vi "Teleop Gears.vi"(11 "Joystick Data":T1) -> ()   [LabVIEW 2013]
uses:
  Joystick Data.ctl
  Gear state.ctl
  <vilib>/Rock Robotics/WPI/Solenoid/WPI_SolenoidValue.ctl
  <vilib>/Rock Robotics/WPI/Solenoid/WPI_SolenoidSetEnum.vi
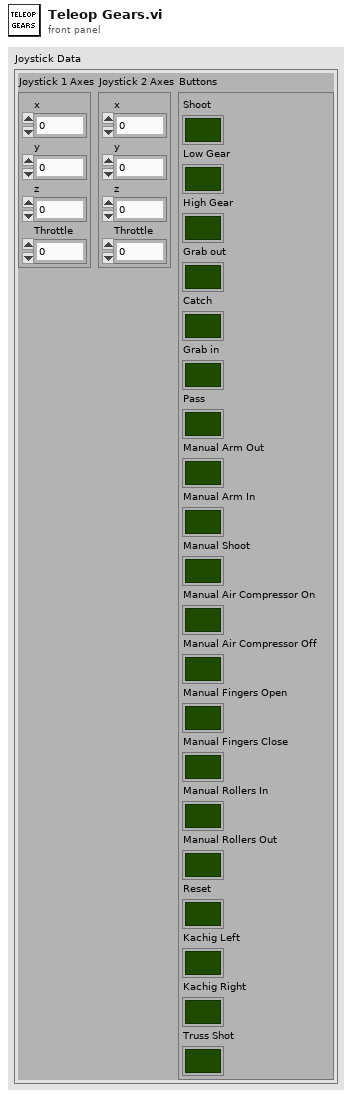
[diagram p1: front panel]
types:
  T1 = typedef "Joystick Data.ctl" = cluster{"Joystick 1 Axes":cluster{"x":dbl, "y":dbl, "z":dbl, "Throttle":dbl}, "Joystick 2 Axes":cluster{"x":dbl, "y":dbl, "z":dbl, "Throttle":dbl}, "Buttons":cluster{"Shoot":bool, "Low Gear":bool, "High Gear":bool, "Grab out":bool, "Catch":bool, "Grab in":bool, "Pass":bool, "Manual Arm Out":bool, "Manual Arm In":bool, "Manual Shoot":bool, "Manual Air Compressor On":bool, "Manual Air Compressor Off":bool, "Manual Fingers Open":bool, "Manual Fingers Close":bool, "Manual Rollers In":bool, "Manual Rollers Out":bool, "Reset":bool, "Kachig Left":bool, "Kachig Right":bool, "Truss Shot":bool}}
  T2 = typedef "Gear state.ctl" = enum16{"idle", "go to low gear", "go to high gear"}
  T3 = typedef "WPI_SolenoidDevRef.ctl" = cluster{"DevStatus":errorcluster, "Solenoid Module":T4, "Forward Solenoid Channel":T5, "Reverse Solenoid Channel":T5}
  T4 = typedef "FPGA_TypedefSolenoidModule.ctl" = enum16{"Solenoid Module 1", "Solenoid Module 2"}
  T5 = typedef "WPI_SolenoidChannel.ctl" = enum8{"Solenoid 1", "Solenoid 2", "Solenoid 3", "Solenoid 4", "Solenoid 5", "Solenoid 6", "Solenoid 7", "Solenoid 8", "Invalid"}
  T6 = typedef "WPI_SolenoidValue.ctl" = enum16{"Off", "On", "Forward", "Reverse"}
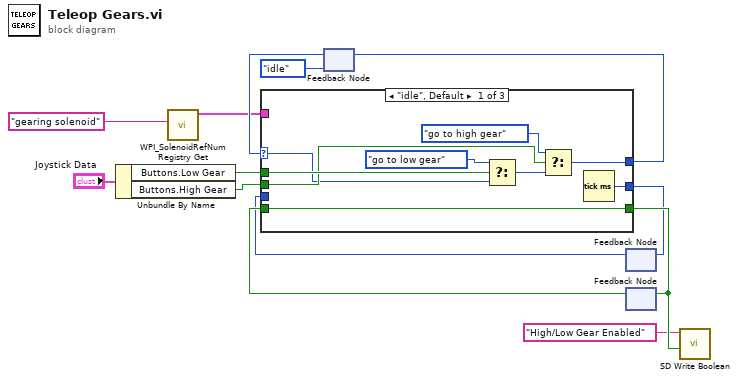
[diagram p0: block diagram]
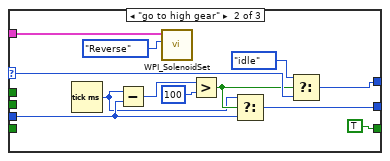
[diagram p2: hidden frame]
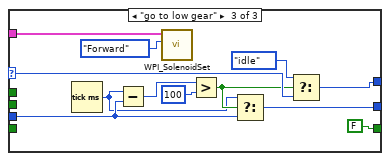
[diagram p3: hidden frame]
diagram:
  n1 = Unbundle By Name("Joystick Data") -> ("Buttons.Low Gear"=w1:bool, "Buttons.High Gear"=w2:bool)
  n2 = call <vilib>:"WPI_SolenoidRefNum Registry Get.vi"("refnum name"="gearing solenoid") -> ("SolenoidDevRef"=w5:T3)  [unwired: 9 in, 1 out]
  n3 = feedback #1(Gear_state."idle") -> (w7:T2)
  n4 = feedback #2() -> (w9:u32)  [unwired: 1 in]
  n5 = feedback #3() -> (w12:bool)  [unwired: 1 in]
  n6 = case shown="\"idle\", Default" w7 {
    selector: w7 -> [w16 w31 w44]
    tunnel: w5 -> [_ w33 w36]
    tunnel: [w19 w24 w43] -> w8
    tunnel: w1 -> [w22 _ _]
    tunnel: w2 -> [w21 _ _]
    tunnel: w9 -> [_ w28 w40]
    tunnel: [w15 w32 w45] -> w10
    tunnel: w12 -> [w14 _ _]
    tunnel: [w14 TRUE FALSE] -> w13
    frame "idle", Default {
      n7 = Select(t=Gear_state."go to low gear", s=w22, f=w16) -> (s? t:f=w20:T2)
      n8 = Select(t=Gear_state."go to high gear", s=w21, f=w20) -> (s? t:f=w19:T2)
      n9 = Tick Count (ms)() -> (millisecond timer value=w15:u32)
    }
    frame "go to high gear" {
      n10 = Tick Count (ms)() -> (millisecond timer value=w27:u32)
      n11 = Subtract(x=w27, y=w28) -> (x-y=w25:u32)
      n12 = call-poly <vilib>:"WPI_SolenoidSet.vi"("Value"=WPI_SolenoidValue."Reverse", "SolenoidDevRef"=w33) -> ()  [unwired: 8 in, 2 out]
      n13 = Greater?(x=w25, y=u32 100 ("x")) -> (0:w29:bool)
      n14 = Select(t=w27, s=w29, f=w28) -> (s? t:f=w32:u32)
      n15 = Select(t=Gear_state."idle", s=w29, f=w31) -> (s? t:f=w24:T2)
    }
    frame "go to low gear" {
      n16 = Tick Count (ms)() -> (millisecond timer value=w39:u32)
      n17 = Subtract(x=w39, y=w40) -> (x-y=w37:u32)
      n18 = call-poly <vilib>:"WPI_SolenoidSet.vi"("Value"=WPI_SolenoidValue."Forward", "SolenoidDevRef"=w36) -> ()  [unwired: 8 in, 2 out]
      n19 = Greater?(x=w37, y=u32 100 ("x")) -> (0:w41:bool)
      n20 = Select(t=w39, s=w41, f=w40) -> (s? t:f=w45:u32)
      n21 = Select(t=Gear_state."idle", s=w41, f=w44) -> (s? t:f=w43:T2)
    }
  }
  n22 = feedback-in #1(w8) -> ()
  n23 = feedback-in #2(w10) -> ()
  n24 = feedback-in #3(w13) -> ()
  n25 = call <vilib>:"SD Write Boolean.vi"("Boolean"=w13, "Name"="High/Low Gear Enabled") -> ()  [unwired: 8 in, 2 out]
